vi "Are Equal.vi"(6 "Tolerance":sgl=1e-06, 10 "Vector 2":refnum<class "Vector 2D.lvclass">, 11 "Vector 1":refnum<class "Vector 2D.lvclass">) -> (3 "Equal":bool)   [LabVIEW 2021, in "Vector 2D.lvclass"]
uses:
  Vector 2D.lvclass
  Vector 2D.lvclass/Vector 2D.ctl
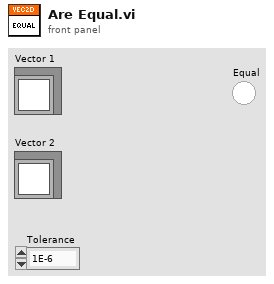
[diagram p1: front panel]
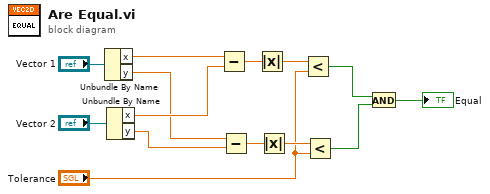
[diagram p0: block diagram]
diagram:
  n1 = Unbundle By Name("Vector 1") -> ("x"=w12:sgl, "y"=w6:sgl)
  n2 = Unbundle By Name("Vector 2") -> ("x"=w11:sgl, "y"=w5:sgl)
  n3 = Subtract(x=w12, y=w11) -> (x-y=w10:sgl)
  n4 = Subtract(x=w6, y=w5) -> (x-y=w7:sgl)
  n5 = Absolute Value(x=w10) -> (abs(x)=w9:sgl)
  n6 = Absolute Value(x=w7) -> (abs(x)=w8:sgl)
  n7 = Less?(x=w9, y="Tolerance") -> (x < y?=w4:bool)
  n8 = Less?(x=w8, y="Tolerance") -> (x < y?=w3:bool)
  n9 = And(x=w4, y=w3) -> (x .and. y?=→"Equal":bool)
